vi "GetI.vi"(8 "error in (no error)":errorcluster, 11 "reference in":refnum<class "GOOP4_Base.lvclass">) -> (0 "error out":errorcluster, 1 "String":string, 2 "i":i32, 3 "reference out":refnum<class "GOOP4_Base.lvclass">)   [LabVIEW 2019, in "GOOP4_Base.lvclass"]
uses:
  GOOP4_Base.lvclass
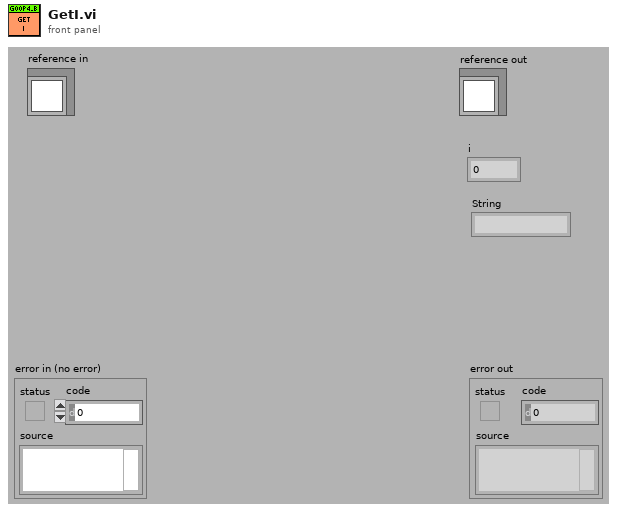
[diagram p1: front panel]
types:
  T1 = typedef "GOOP4_Base.lvclass/ObjectAttributes.ctl" = cluster{"i":i32}
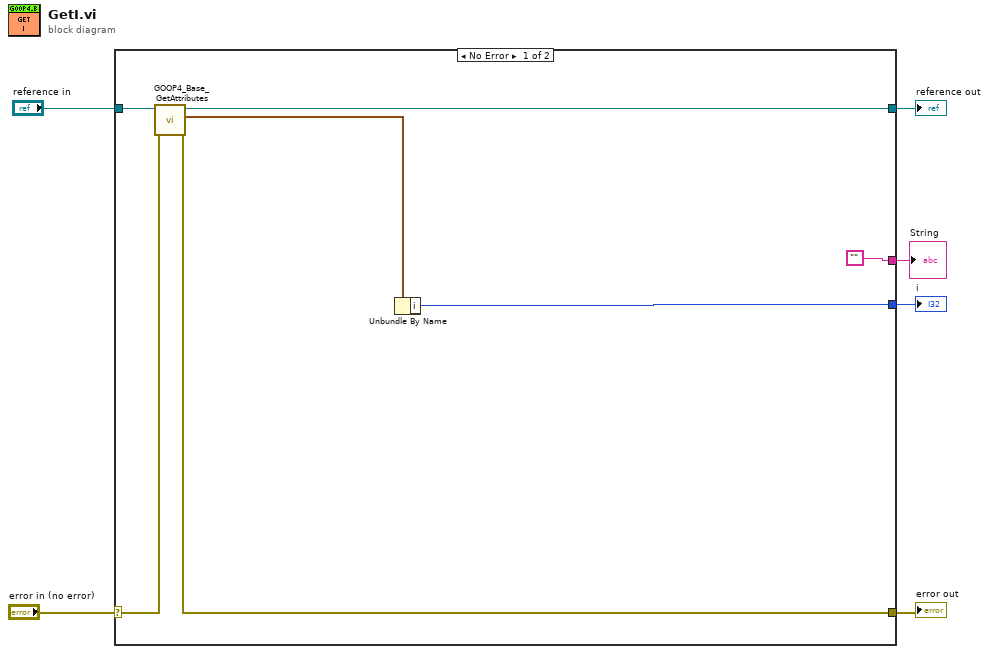
[diagram p0: block diagram]
diagram:
  n1 = case shown="No Error" "error in (no error)" {
    selector: "error in (no error)" -> [w13 w15]
    tunnel: [w11 w15] -> w5
    tunnel: [w9 w14] -> w3
    tunnel: "reference in" -> [w10 w14]
    tunnel: [w8 _] -> w2
    tunnel: ["" _] -> w1
    frame No Error {
      n2 = call "GOOP4_Base_GetAttributes.vi"("error in (no error)"=w13, "reference in"=w10) -> ("error out"=w11:errorcluster, "Data"=w12:T1, "reference out"=w9:refnum<class "GOOP4_Base.lvclass">)  [unwired: 6 in, 1 out]
      n3 = Unbundle By Name(w12) -> ("i"=w8:i32)
    }
    frame Error {
    }
  }
  "error out" <- w5
  "reference out" <- w3
  "i" <- w2
  "String" <- w1
